vi "Trim End.vi"(8 "error in (no error)":errorcluster, 10 "String":string, 11 "ProtoParser in":refnum<class "ProtoParser.lvclass">) -> (0 "error out":errorcluster, 2 "Trimmed":string, 3 "ProtoParser out":refnum<class "ProtoParser.lvclass">)   [LabVIEW 2020, in "LV-Protoc.lvlib" / "ProtoParser.lvclass"]
uses:
  ProtoParser.lvclass
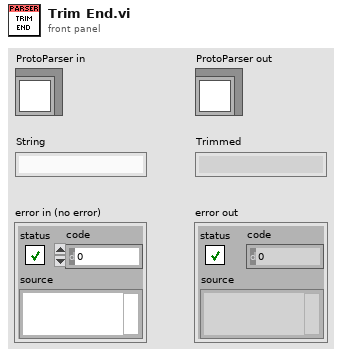
[diagram p1: front panel]
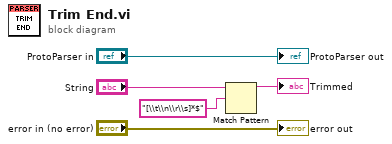
[diagram p0: block diagram]
diagram:
  n1 = Match Pattern(string="String", regular expression="[\\t\\n\\r\\s]*$") -> (before substring=→"Trimmed":string)  [unwired: 1 in, 3 out]
  "error out" <- "error in (no error)"
  "ProtoParser out" <- "ProtoParser in"
